vi "Check_EnFlo_Tunnel_Cond.vi"() -> (0 "Status Cluster":T1, 1 "Heaters On?":bool)   [LabVIEW 2014]
uses:
  Anemometry/Anemometry Sub Vis/Gen Trav/Status_Cluster.ctl
  Anemometry/Anemometry Sub Vis/Gen Trav/Multi_Run_Status.ctl
  Anemometry/Anemometry Sub Vis/Controls/In_Range.ctl
  Anemometry/Anemometry Sub Vis/Globals/Meas_global.vi
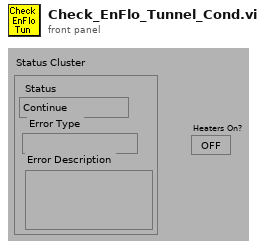
[diagram p1: front panel]
types:
  T1 = typedef "Status_Cluster.ctl" = cluster{"Status":T2, "Error Type":string, "Error Description":string}
  T2 = typedef "Multi_Run_Status.ctl" = enum16{"Continue", "Jump to Next Point", "Jump to Next Row", "Jump To Fall Back", "Terminate Run"}
  T3 = typedef "In_Range.ctl" = enum16{"%", "±", "% & ±"}
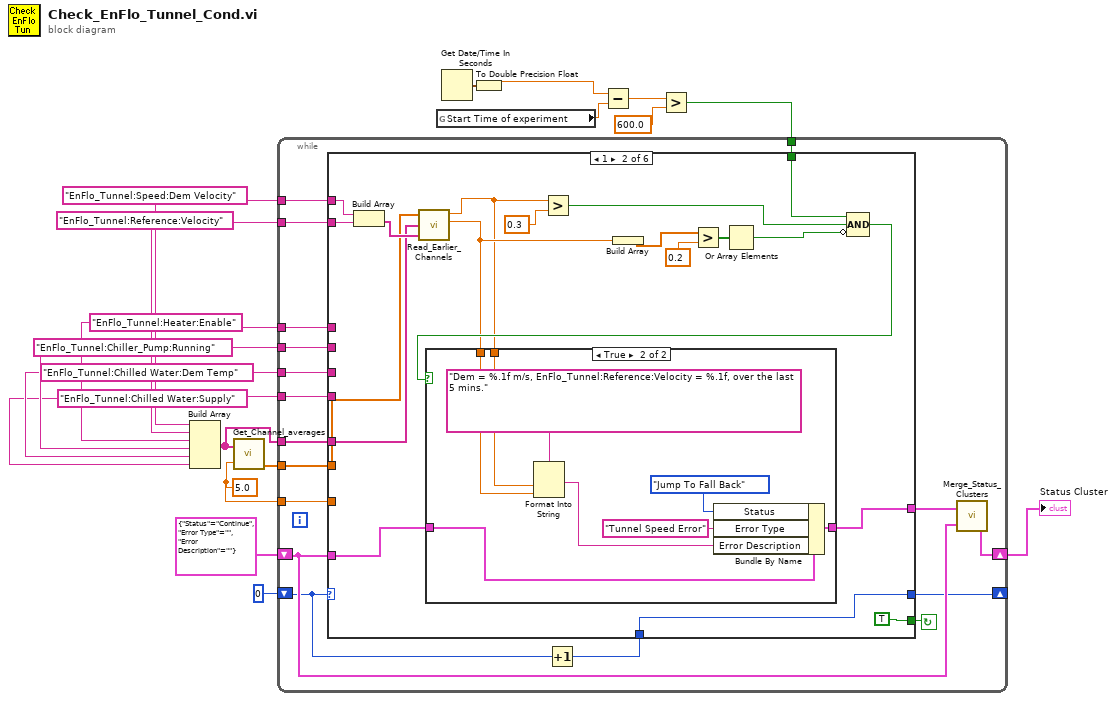
[diagram p0: block diagram]
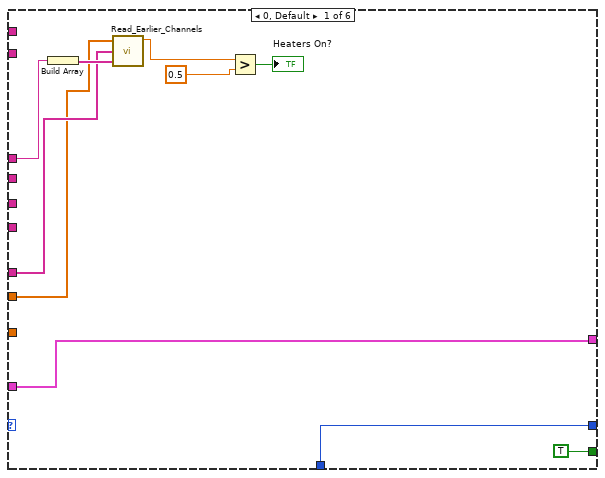
[diagram p2: hidden frame]
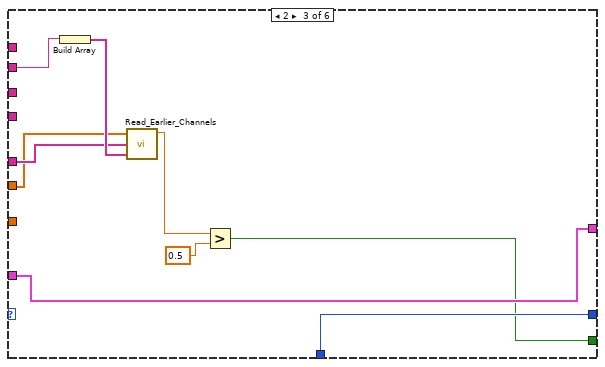
[diagram p4: hidden frame]
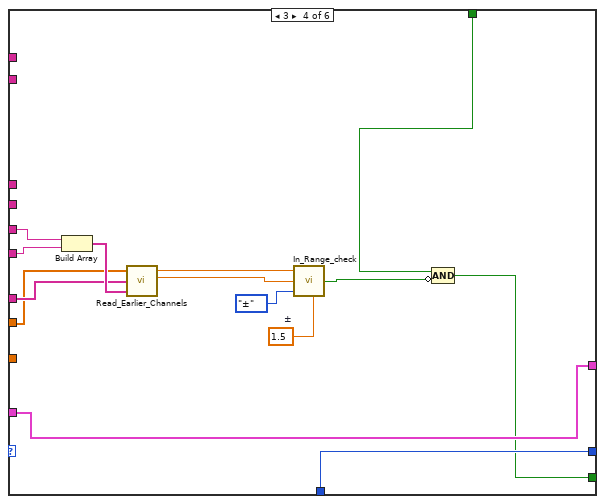
[diagram p5: hidden frame]
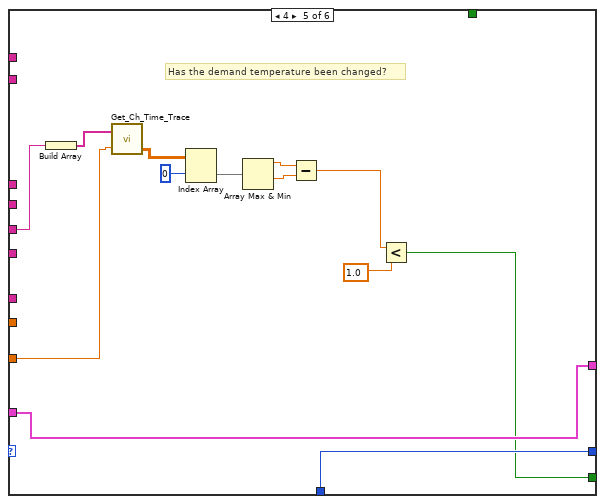
[diagram p6: hidden frame]
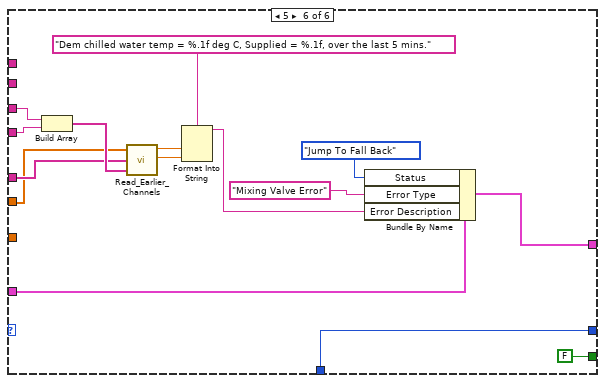
[diagram p7: hidden frame]
diagram:
  w8 = "EnFlo_Tunnel:Chilled Water:Supply"
  w9 = "EnFlo_Tunnel:Chilled Water:Dem Temp"
  w10 = "EnFlo_Tunnel:Chiller_Pump:Running"
  w15 = "EnFlo_Tunnel:Heater:Enable"
  w1 = 5.0 ("Averaging time (mins)")
  w17 = "EnFlo_Tunnel:Speed:Dem Velocity"
  w16 = "EnFlo_Tunnel:Reference:Velocity"
  n1 = Build Array(w17, w16, w15, w10, w9, w8) -> (w12:string[])
  n2 = call "Get_Channel_averages.vi"("Desired Ch Names"=w12, "Averaging time (mins)"=w1) -> ("number"=w18:dbl[])  [unwired: 1 in, 2 out]
  n3 = global read "Meas_global.vi" "Start Time of experiment"() -> (w5:dbl)
  n4 = Get Date/Time In Seconds() -> (seconds since 1Jan1904=w2:timestamp)
  n5 = To Double Precision Float(number=w2) -> (double precision float=w4:dbl)
  n6 = Subtract(x=w4, y=w5) -> (x-y=w6:dbl)
  n7 = Greater?(x=w6, y=600.0) -> (0:w3:bool)
  n8 = while {
    tunnel: w3 -> [w20]
    tunnel: w8 -> [w21]
    tunnel: w9 -> [w22]
    tunnel: w10 -> [w23]
    shift-left: 0 -> [w26]
    shift-right: [w25] -> _
    tunnel: w15 -> [w30]
    tunnel: w16 -> [w31]
    tunnel: w17 -> [w32]
    tunnel: w12 -> [w33]
    tunnel: w18 -> [w34]
    shift-left: T1 {"Status"=enum."Continue", "Error Type"="", "Error Description"=""} ("Status Cluster In") -> [w28]
    shift-right: [w27] -> w14
    tunnel: w1 -> [w19]
    stop <- w35 continue-if-true
    n9 = Increment(x=w26) -> (x+1=w24:i32)
    n10 = case shown="1" w26 {
      tunnel: [TRUE TRUE w75 w83 w105 FALSE] -> w35
      tunnel: w34 -> [w40 w55 w79 w93 _ w122]
      tunnel: w33 -> [w41 w56 w80 w94 _ w123]
      tunnel: w32 -> [_ w59 _ _ _ _]
      tunnel: w31 -> [_ w58 _ _ _ _]
      tunnel: w28 -> [w45 w63 w82 w96 w109 w111]
      tunnel: [w45 w61 w82 w96 w109 w110] -> w29
      tunnel: w30 -> [w38 _ _ _ _ _]
      tunnel: w24 -> [w39 w47 w78 w92 w108 w121]
      tunnel: [w39 w47 w78 w92 w108 w121] -> w25
      tunnel: w23 -> [_ _ w77 _ _ _]
      tunnel: w22 -> [_ _ _ w91 w104 w119]
      tunnel: w21 -> [_ _ _ w90 _ w120]
      tunnel: w20 -> [_ w46 _ w84 _ _]
      tunnel: w19 -> [_ _ _ _ w102 _]
      frame 0, Default {
        n11 = Build Array(w38) -> (w42:string[])
        n12 = call "Read_Earlier_Channels.vi"("Present scan array"=w40, "Ch names"=w41, "Desired Channels"=w42) -> ("Index 0"=w37:dbl)  [unwired: 5 out]
        n13 = Greater?(x=w37, y=0.5) -> (0:→"Heaters On?":bool)
      }
      frame 1 {
        n14 = Build Array(w59, w58) -> (w57:string[])
        n15 = call "Read_Earlier_Channels.vi"("Present scan array"=w55, "Ch names"=w56, "Desired Channels"=w57) -> ("Index 0"=w53:dbl, "Index 1"=w54:dbl)  [unwired: 4 out]
        n16 = Greater?(x=w53, y=0.3) -> (0:w48:bool)
        n17 = Build Array(w54) -> (w51:dbl[])
        n18 = Greater?(x=w51, y=0.2) -> (0:w49:bool[])
        n19 = Or Array Elements(Boolean array=w49) -> (logical OR=w62:bool)
        n20 = Compound Arithmetic op=AND(w46, w48, invert w62) -> (w60:bool)
        n21 = case shown="True" w60 {
          tunnel: [w65 w72] -> w61
          tunnel: w63 -> [w65 w73]
          tunnel: w53 -> [_ w67]
          tunnel: w54 -> [_ w66]
          frame False {
          }
          frame True {
            n22 = Format Into String(format string="Dem = %.1f m/s, EnFlo_Tunnel:Reference:Velocity = %.1f, over the last 5 mins." ("Format String"), w67, w66) -> (resulting string=w68:string)  [unwired: 2 in, 1 out]
            n23 = Bundle By Name(cluster=w73, "Status"=Multi_Run_Status."Jump To Fall Back", "Error Type"="Tunnel Speed Error" ("Bundle Element"), "Error Description"=w68) -> (w72:T1)
          }
        }
      }
      frame 2 {
        n24 = Build Array(w77) -> (w81:string[])
        n25 = call "Read_Earlier_Channels.vi"("Present scan array"=w79, "Ch names"=w80, "Desired Channels"=w81) -> ("Index 0"=w74:dbl)  [unwired: 5 out]
        n26 = Greater?(x=w74, y=0.5) -> (0:w75:bool)
      }
      frame 3 {
        w87 = 1.5  # ±
        n27 = Build Array(w91, w90) -> (w95:string[])
        n28 = call "Read_Earlier_Channels.vi"("Present scan array"=w93, "Ch names"=w94, "Desired Channels"=w95) -> ("Index 0"=w89:dbl, "Index 1"=w88:dbl)  [unwired: 4 out]
        n29 = call "In_Range_check.vi"("±"=w87, "Mode"=In_Range."±", "Value"=w88, "Setpoint"=w89) -> ("In Range"=w85:bool)  [unwired: 1 in, 2 out]
        n30 = Compound Arithmetic op=AND(w84, invert w85) -> (w83:bool)
      }
      frame 4 {
        # "Has the demand temperature been changed?"
        n31 = Build Array(w104) -> (w103:string[])
        n32 = call "Get_Ch_Time_Trace.vi"("Desired Ch Names"=w103, "History Length (mins)"=w102) -> ("Output array"=w101:dbl[][])  [unwired: 2 out]
        n33 = Index Array(array=w101, index (row)=0 ("Index")) -> (element=w100:dbl[])  [unwired: 1 in]
        n34 = Array Max & Min(array=w100) -> (max value=w99:dbl, min value=w98:dbl)  [unwired: 2 out]
        n35 = Subtract(x=w99, y=w98) -> (x-y=w97:dbl)
        n36 = Less?(x=w97, y=1.0) -> (x < y?=w105:bool)
      }
      frame 5 {
        n37 = Build Array(w119, w120) -> (w124:string[])
        n38 = call "Read_Earlier_Channels.vi"("Present scan array"=w122, "Ch names"=w123, "Desired Channels"=w124) -> ("Index 0"=w113:dbl, "Index 1"=w112:dbl)  [unwired: 4 out]
        n39 = Format Into String(format string="Dem chilled water temp = %.1f deg C, Supplied = %.1f, over the last 5 mins." ("Format String"), w113, w112) -> (resulting string=w114:string)  [unwired: 2 in, 1 out]
        n40 = Bundle By Name(cluster=w111, "Status"=Multi_Run_Status."Jump To Fall Back", "Error Type"="Mixing Valve Error" ("Bundle Element"), "Error Description"=w114) -> (w110:T1)
      }
    }
    n41 = call "Merge_Status_Clusters.vi"("Status Cluster 2"=w28, "Status Cluster 1"=w29) -> ("Status Cluster Out"=w27:T1)
  }
  "Status Cluster" <- w14
